vi "BotSpeakSerial_WriteRead_test.vi"(0 "error In":errorcluster, 1 "To Write":string, 2 "Connection In":T1) -> (3 "error out":errorcluster, 4 "Reply":string, 5 "Reply EOF":string, 6 "Connection Out":T1)   [LabVIEW 2012]
uses:
  <userlib>/BotSpeak/VIs/SubVIs/CommState.ctl
  <userlib>/BotSpeak/VIs/Direct/BotSpeak_Control.ctl
  <userlib>/BotSpeak/VIs/SubVIs/BotSpeak_Globals.vi
panel:
  out "Buffer":u32[](graph)
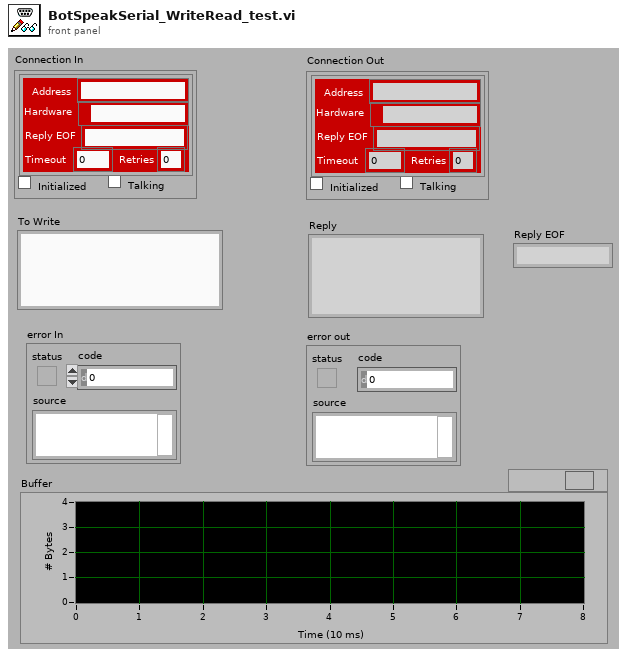
[diagram p1: front panel]
types:
  T1 = typedef "CommState.ctl" = cluster{"Bot Settings":T2, "Initialized":bool, "Talking":bool}
  T2 = typedef "BotSpeak_Control.ctl" = cluster{"Address":string, "Reply EOF":string, "Hardware":path, "Retries":i8, "Timeout":i32}
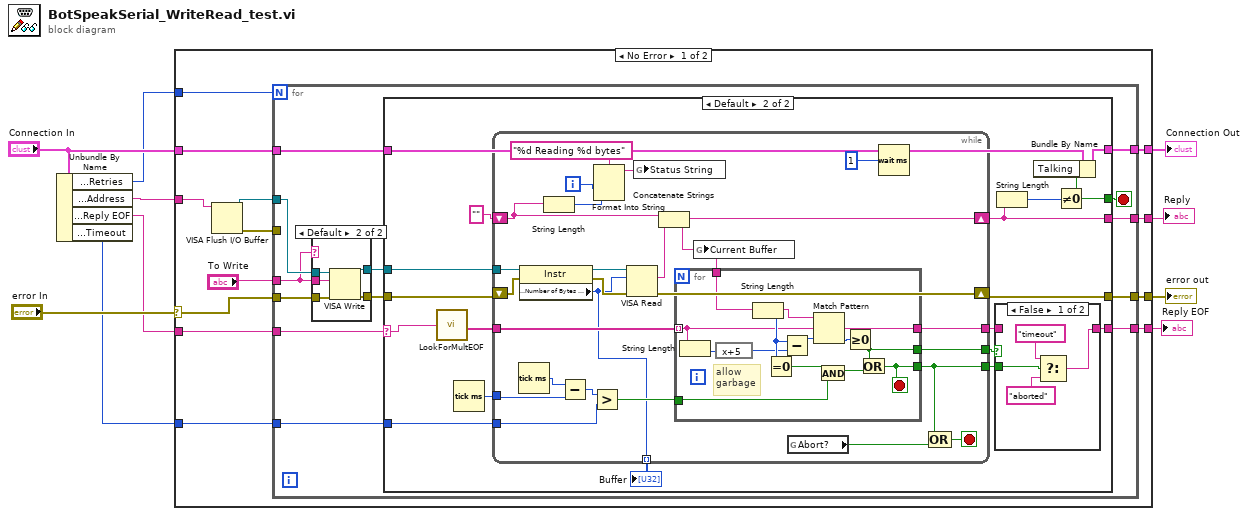
[diagram p0: block diagram]
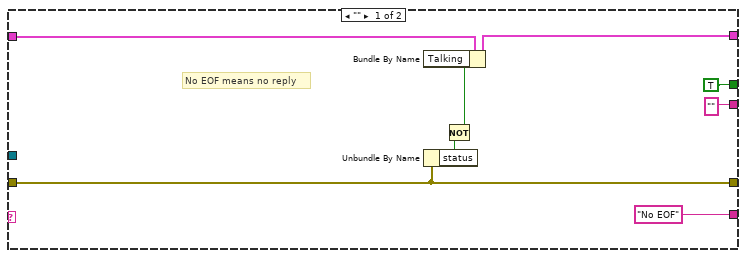
[diagram p3: hidden frame]
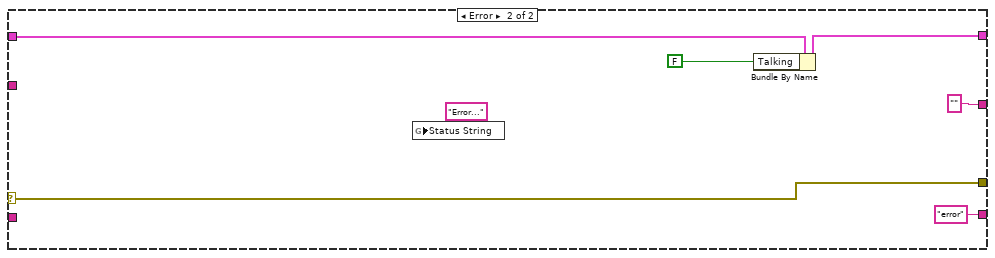
[diagram p5: hidden frame]
diagram:
  n1 = Unbundle By Name("Connection In") -> ("Bot Settings.Retries"=w4:i8, "Bot Settings.Address"=w5:string, "Bot Settings.Reply EOF"=w2:string, "Bot Settings.Timeout"=w3:i32)
  n2 = case shown="No Error" "error In" {
    selector: "error In" -> [w15 w113]
    tunnel: [w23 ""] -> w7
    tunnel: [w22 w113] -> w8
    tunnel: "Connection In" -> [w21 w117]
    tunnel: [w20 w115] -> w9
    tunnel: w4 -> [w19 _]
    tunnel: w5 -> [w13 _]
    tunnel: w3 -> [w18 _]
    tunnel: w2 -> [w16 _]
    tunnel: [w14 "error" ("Reply EOF")] -> w1
    frame No Error {
      n3 = VISA Flush I/O Buffer(VISA resource name=w13) -> (VISA resource name out=w12:refnum<visa-resource-name>, error out=w11:errorcluster)  [unwired: 2 in]
      n4 = for {
        N: w19 -> [_]
        tunnel: "To Write" -> [w24]
        tunnel: [w36] -> w23
        tunnel: [w31] -> w22
        tunnel: w15 -> [w35]
        tunnel: w21 -> [w29]
        tunnel: [w32] -> w20
        tunnel: w18 -> [w28]
        tunnel: w16 -> [w27]
        tunnel: w12 -> [w26]
        tunnel: [w25] -> w14
        tunnel: w11 -> [_]
        stop <- w30 stop-if-true
        n5 = case shown="Default" w24 {
          tunnel: w24 -> [_ w43]
          tunnel: w35 -> [w38 w42]
          tunnel: [w37 w41] -> w34
          tunnel: [w38 w40] -> w33
          tunnel: w26 -> [w37 w39]
          frame "" {
          }
          frame Default {
            n6 = VISA Write(VISA resource name=w39, write buffer=w43, error in (no error)=w42) -> (VISA resource name out=w41:refnum<visa-resource-name>, error out=w40:errorcluster)  [unwired: 1 out]
          }
        }
        n7 = case shown="Default" w27 {
          selector: w27 -> [_ w52]
          tunnel: ["" w62] -> w36
          tunnel: [w47 w63] -> w31
          tunnel: w34 -> [_ w68]
          tunnel: w33 -> [w47 w67]
          tunnel: w29 -> [w48 w65]
          tunnel: [w46 w64] -> w32
          tunnel: [TRUE w54] -> w30
          tunnel: w28 -> [_ w60]
          tunnel: ["No EOF" ("Reply EOF") w56] -> w25
          frame "" {
            # "No EOF means no reply"
            n8 = Unbundle By Name(w47) -> ("status"=w50:bool)
            n9 = Not(x=w50) -> (.not. x?=w49:bool)
            n10 = Bundle By Name(cluster=w48, "Talking"=w49) -> (w46:T1)
          }
          frame Default {
            n11 = call <userlib>:"LookForMultEOF.vi"("Reply EOF"=w52) -> ("Array"=w59:string[])
            n12 = Tick Count (ms)() -> (millisecond timer value=w66:u32)
            n13 = while {
              tunnel: w59 -> [w94]
              shift-right: [w99] -> w63
              shift-left: w67 -> [w98]
              shift-right: [w81] -> w62
              shift-left: "" -> [w84]
              tunnel: w68 -> [w93]
              tunnel: w66 -> [w88]
              tunnel: w60 -> [w79]
              tunnel: [w77] -> w58
              tunnel: [w78] -> w57
              tunnel: [w76] -> w55
              tunnel: [w75] -> w53 mode=indexing
              i -> [w86]
              stop <- w90 stop-if-true
              n14 = Tick Count (ms)() -> (millisecond timer value=w89:u32)
              n15 = property class="Instr"(reference=w93, error in=w98) -> (reference out=w97:refnum<visa-resource-name>, error out=w96:errorcluster, "Serial Settings:Number of Bytes at Serial Port"=w75:u32)
              n16 = String Length(string=w84) -> (length=w83:i32)
              n17 = Subtract(x=w89, y=w88) -> (x-y=w92:u32)
              n18 = Greater?(x=w92, y=w79) -> (0:w91:bool)
              n19 = Format Into String(format string="%d Reading %d bytes", w86, w83) -> (resulting string=w85:string)  [unwired: 2 in, 1 out]
              n20 = VISA Read(VISA resource name=w97, byte count=w75, error in (no error)=w96) -> (read buffer=w95:string, error out=w99:errorcluster)  [unwired: 2 out]
              n21 = global write "BotSpeak_Globals.vi" "Status String"(w85) -> ()
              n22 = Concatenate Strings(w84, w95) -> (w81:string)
              n23 = for {
                tunnel: w94 -> [w103] mode=indexing
                tunnel: w91 -> [w110]
                tunnel: w81 -> [w101]
                tunnel: [w104] -> w76
                tunnel: [w103] -> w78
                tunnel: [w102] -> w77
                stop <- w104 stop-if-true
                # "allow\ngarbage"
                n24 = String Length(string=w103) -> (length=w108:i32)
                n25 = expression code="x+5"(w108) -> (w100:i32)
                n26 = String Length(string=w101) -> (length=w106:i32)
                n27 = Equal To 0?(x=w106) -> (x = 0?=w109:bool)
                n28 = Subtract(x=w106, y=w100) -> (x-y=w107:i32)
                n29 = Match Pattern(string=w101, regular expression=w103, offset (0)=w107) -> (offset past match=w111:i32)  [unwired: 3 out]
                n30 = And(x=w109, y=w110) -> (x .and. y?=w105:bool)
                n31 = Greater Or Equal To 0?(x=w111) -> (x >= 0?=w102:bool)
                n32 = Or(x=w102, y=w105) -> (x .or. y?=w104:bool)
              }
              n33 = global write "BotSpeak_Globals.vi" "Current Buffer"(w81) -> ()
              n34 = global read "BotSpeak_Globals.vi" "Abort?"() -> (w80:bool)
              n35 = Wait (ms)(milliseconds to wait=u32 1) -> ()  [unwired: 1 out]
              n36 = Compound Arithmetic op=OR(w76, w80) -> (w90:bool)
            }
            "Buffer" <- w53
            n37 = case shown="False" w58 {
              tunnel: w57 -> [_ w74]
              tunnel: [w70 w74] -> w56
              tunnel: w55 -> [w72 _]
              frame False {
                n38 = Select(t="timeout" ("Reply EOF"), s=w72, f="aborted" ("Reply EOF")) -> (s? t:f=w70:string)
              }
              frame True {
              }
            }
            n39 = String Length(string=w62) -> (length=w61:i32)
            n40 = Not Equal To 0?(x=w61) -> (x != 0?=w54:bool)
            n41 = Bundle By Name(cluster=w65, "Talking"=w54) -> (w64:T1)
          }
        }
      }
    }
    frame Error {
      n42 = global write "BotSpeak_Globals.vi" "Status String"("Error..." ("Status String")) -> ()
      n43 = Bundle By Name(cluster=w117, "Talking"=FALSE) -> (w115:T1)
    }
  }
  "Connection Out" <- w9
  "error out" <- w8
  "Reply" <- w7
  "Reply EOF" <- w1
